vi "New 1ch.vi"(0 "VISA resource name out":refnum<visa-resource-name>, 9 "Number of channels":i32, 11 "error out":errorcluster) -> (3 "VISA resource name out 2":refnum<visa-resource-name>, 4 "Array 2":dbl[](array[numeric]), 6 "Array":dbl[](array[numeric]), 15 "error out 2":errorcluster)   [LabVIEW 2015]
uses:
  <instrlib>/Keithley 27XX/Public/Data/Read Multiple Direct.vi
  <instrlib>/Keithley 27XX/Keithley 27XX.lvlib
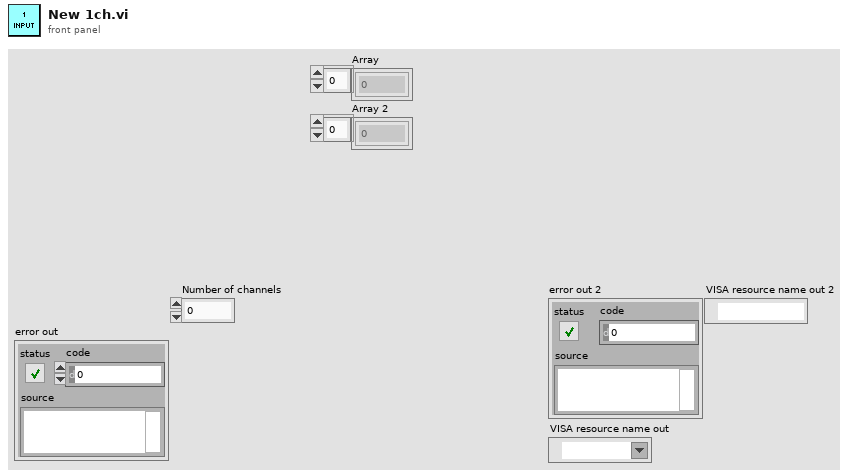
[diagram p1: front panel]
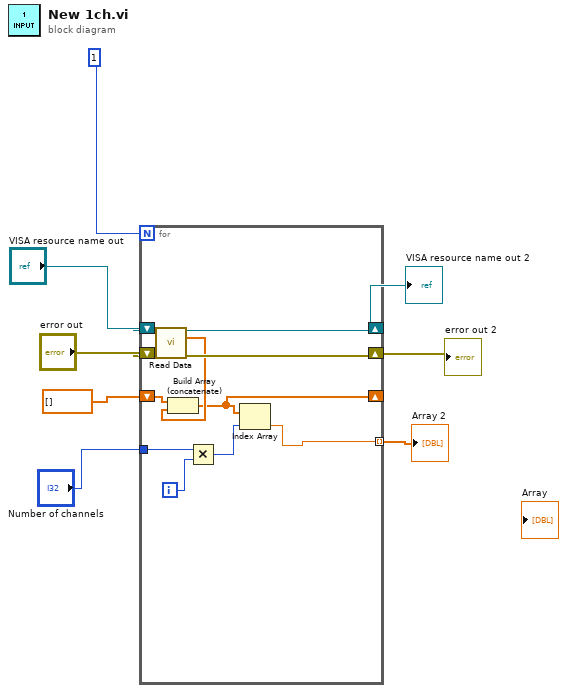
[diagram p0: block diagram]
diagram:
  n1 = for {
    N: 1 -> [_]
    shift-right: [w18] -> w7
    shift-left: "VISA resource name out" -> [w17]
    shift-right: [w19] -> w8
    shift-left: "error out" -> [w16]
    shift-right: [w10] -> _
    shift-left: dbl[] [] -> [w15]
    tunnel: "Number of channels" -> [w12]
    tunnel: [w9] -> w1 mode=indexing
    i -> [w13]
    n2 = call-poly <instrlib>:"Read Data.vi"("VISA resource name"=w17, "error in (no error)"=w16) -> ("VISA resource name out"=w18:refnum<visa-resource-name>, "Measurement Data"=w14:dbl[], "error out"=w19:errorcluster)  [unwired: 8 in, 3 out]
    n3 = Build Array (concatenate)(w15, w14) -> (w10:dbl[])
    n4 = Multiply(x=w12, y=w13) -> (x*y=w11:i32)
    n5 = Index Array(array=w10, index=w11) -> (element=w9:dbl)
  }
  "error out 2" <- w8
  "VISA resource name out 2" <- w7
  "Array 2" <- w1
